vi "processUseControlBodyOnlyFlag_start.vi"(7 "useControlBodyOnly":bool, 8 "error in (no error)":errorcluster, 11 "refList":refnum<vi>[](array[refnum])) -> (0 "error out":errorcluster, 3 "refList(dup)":refnum<vi>[](array[refnum]), 4 "LabelVisibilityList":bool[](array[boolean]), 6 "captionVisibilityList":bool[](array[boolean]))   [LabVIEW 2023]
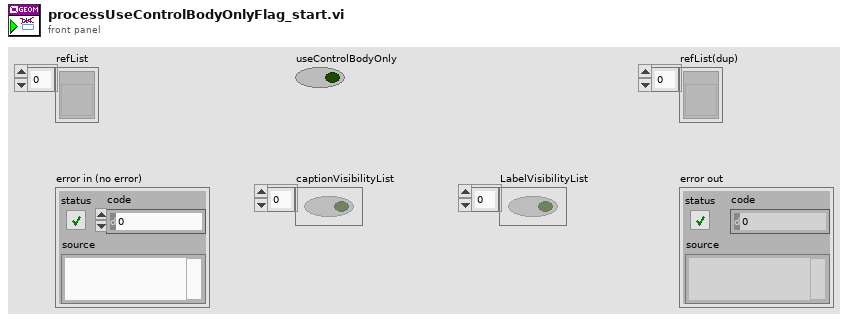
[diagram p1: front panel]
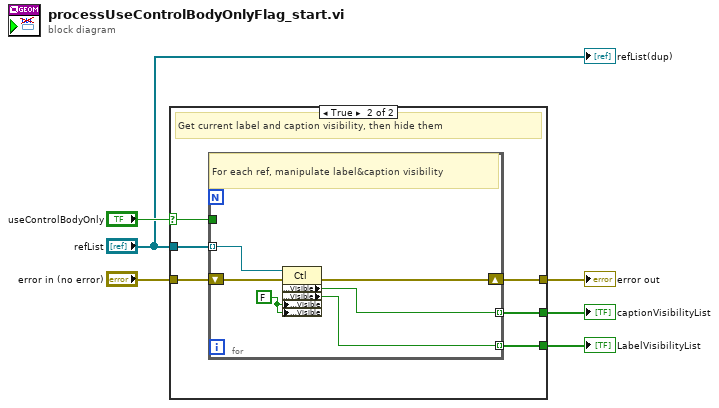
[diagram p0: block diagram]
diagram:
  n1 = case shown="True" "useControlBodyOnly" {
    selector: "useControlBodyOnly" -> [_ w11]
    tunnel: "error in (no error)" -> [w7 w13]
    tunnel: [w7 w12] -> w3
    tunnel: [_ w10] -> w5
    tunnel: [_ w9] -> w6
    tunnel: "refList" -> [_ w8]
    frame False {
      # "Nothing to do"
    }
    frame True {
      # "Get current label and caption visibility, then hide them"
      n2 = for {
        tunnel: w8 -> [w19] mode=indexing
        shift-right: [w17] -> w12
        shift-left: w13 -> [w18]
        tunnel: w11 -> [_]
        tunnel: [w16] -> w10 mode=indexing
        tunnel: [w15] -> w9 mode=indexing
        w14 = FALSE ("Caption.Visible")
        # "For each ref, manipulate label&caption visibility"
        n3 = property class="Ctl"(reference=w19, error in=w18, "Caption.Visible"=w14, "Label.Visible"=w14) -> (error out=w17:errorcluster, "Caption.Visible"=w16:bool, "Label.Visible"=w15:bool)  [unwired: 1 out]
      }
    }
  }
  "LabelVisibilityList" <- w6
  "captionVisibilityList" <- w5
  "error out" <- w3
  "refList(dup)" <- "refList"
